vi "setup_serial.vi"(0 "COM Port":refnum<visa-resource-name>) -> (1 "error out":errorcluster, 2 "VISA resource name out":refnum<visa-resource-name>)   [LabVIEW 2015]
uses:
  <vilib>/Instr/_visa.llb/VISA Configure Serial Port (Instr).vi
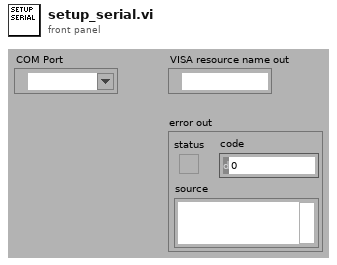
[diagram p1: front panel]
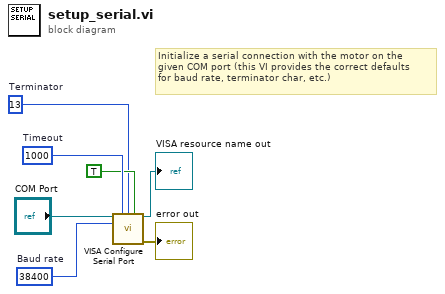
[diagram p0: block diagram]
diagram:
  w4 = u32 1000  # Timeout
  w2 = u32 38400  # Baud rate
  w1 = u8 13  # Terminator
  # "Initialize a serial connection with the motor on the\ngiven COM port (this VI provides the correct defaults\nfor baud rate, terminator char, etc.)"
  n1 = call-poly "VISA Configure Serial Port"("VISA resource name"="COM Port", "timeout (10sec)"=w4, "termination char\n(0xA = '\\n' = LF)"=w1, "Enable Termination\nChar (T)"=TRUE, "baud rate (9600)"=w2) -> ("VISA resource name out"=→"VISA resource name out":refnum<visa-resource-name>, "error out"=→"error out":errorcluster)  [unwired: 9 in]
